vi "Bug2Test.vi"() -> ()   [LabVIEW 2013]
doc: "This example continually replans a path from Start to Goal while following the best known path, including through obstacles if necessary.\nThe Anytime D* search algorithm is useful when the world or the robot's understanding of the world is changing. Anytime D* maintains more information than the A* search algorithm so the robot can backtrack and find a new path more easily if it discovers the original path will not work."
panel:
  in  "Loop Time":u32=100
  out "Current Y":i32
  out "Current X":i32
  in  "y Goal":i32
  in  "x Goal":i32
  in  "Random Obstacles?":bool
  in  "% Random Obstacles":dbl=40.0 min=0.0 max=100.0 step=1.0 format="%#_3g"
  out "path on obstacles":dbl[][](graph)
  in  "y start":i32
  in  "x start":i32
  # "Configuration"
  # "X"
  # "Y"
  # "Start"
  # "X"
  # "Y"
  # "Goal"
  # "1) Choose the Start and Goal location and the % Random Obstacles.\n2) Run the VI.\n3) Adjust the controls in the Run-time Controls section to see the \n     effect each option has on path planning\n4) Change the Run Mode to Single Step to pause after each time\n the AD* VI runs"
  # "Robot"
  # "Obstacle"
  # "Unknown"
  # "Free"
  # "Path"
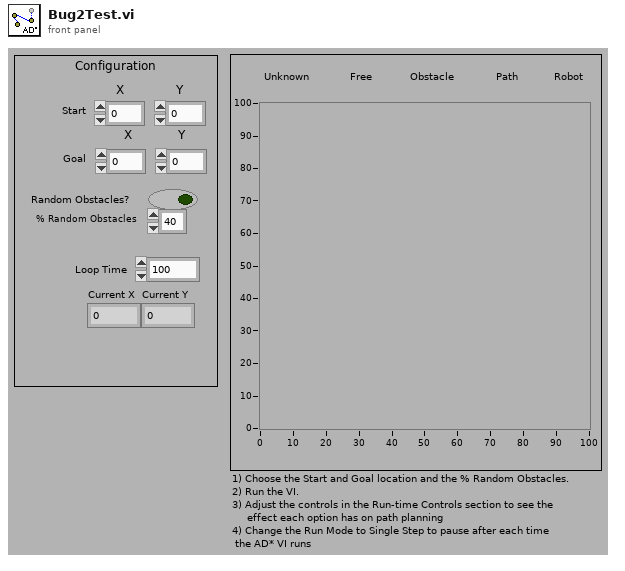
[diagram p1: front panel]
types:
  T1 = cluster{"x start":i32, "y start":i32, "x Goal":i32, "y Goal":i32}
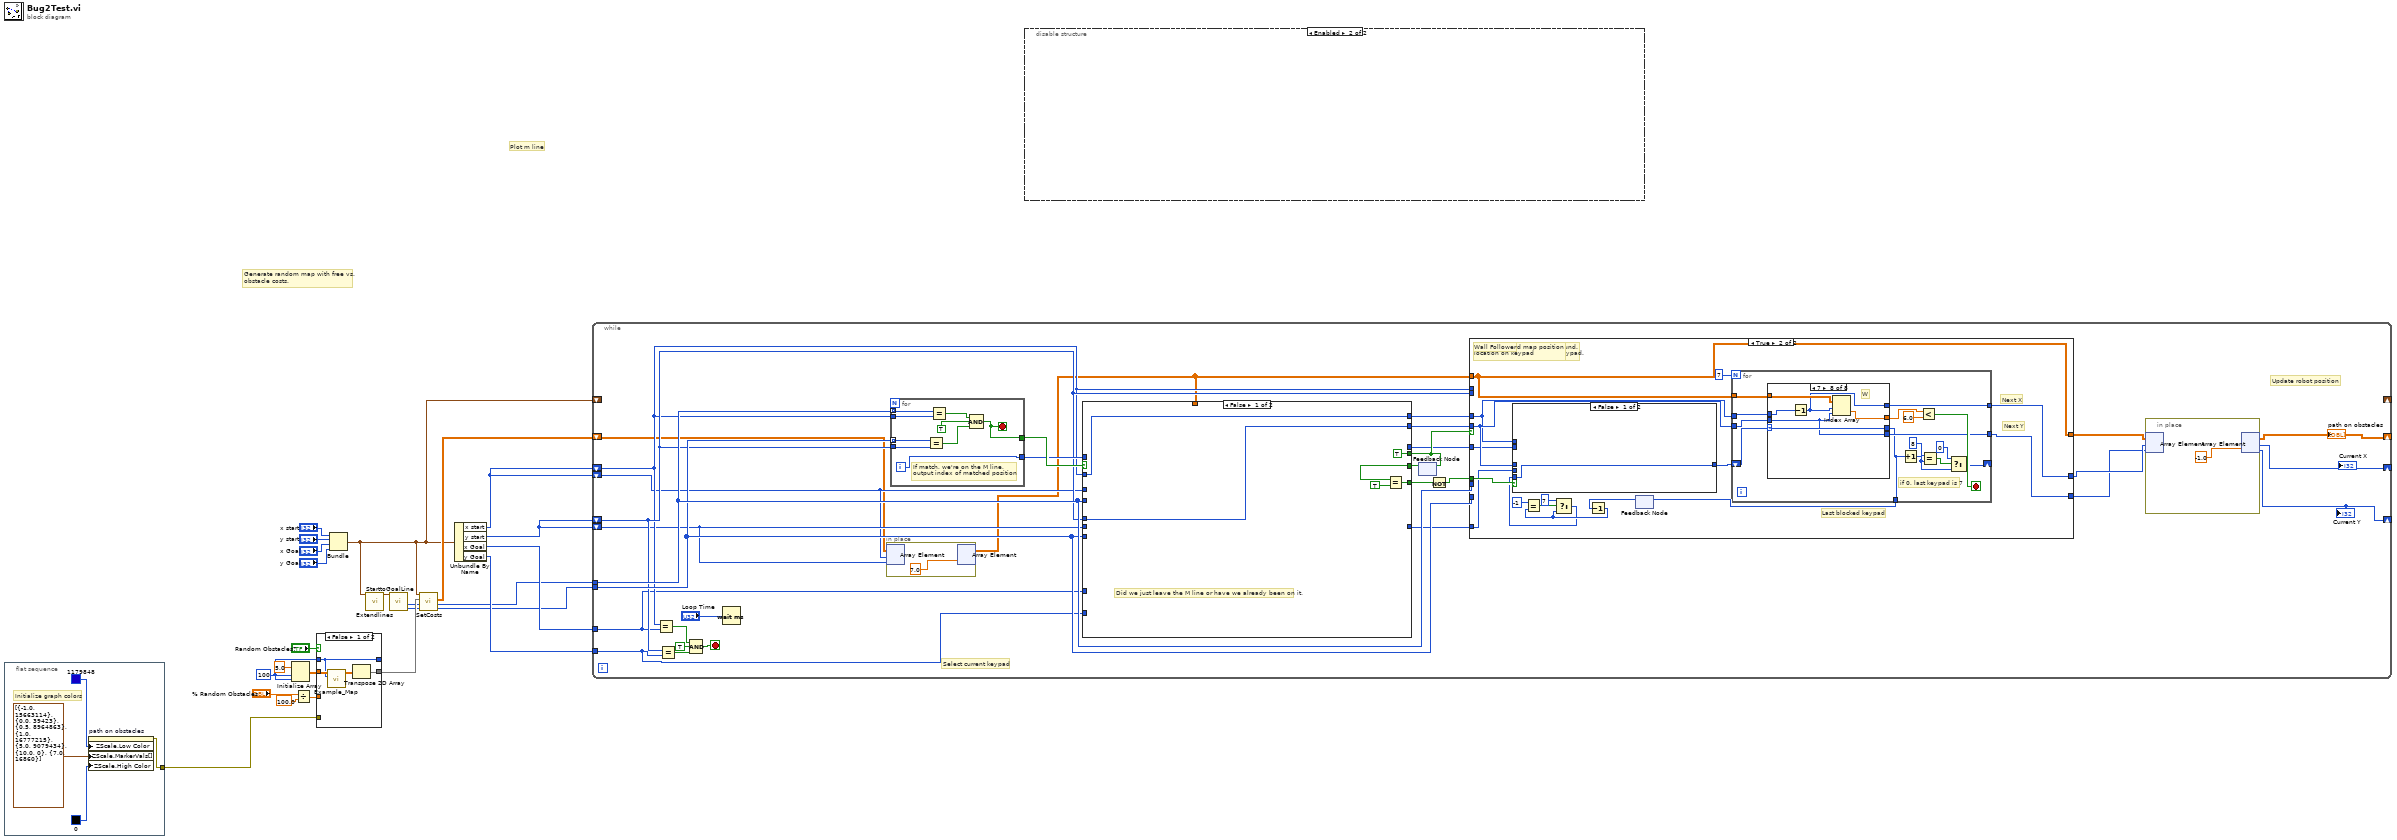
[diagram p0: block diagram]
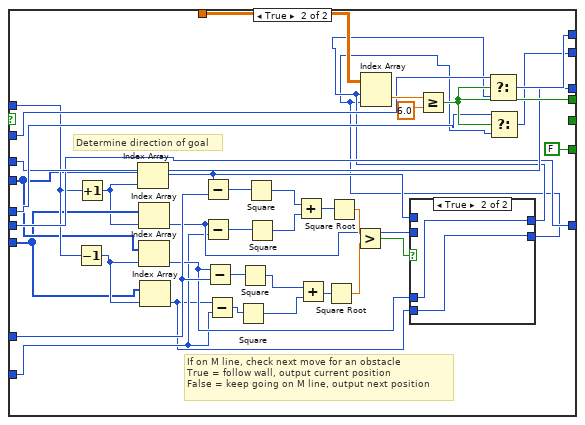
[diagram p2: hidden frame]
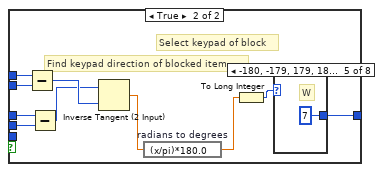
[diagram p5: hidden frame]
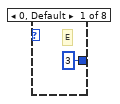
[diagram p6: hidden frame]
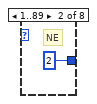
[diagram p7: hidden frame]
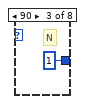
[diagram p8: hidden frame]
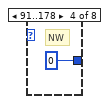
[diagram p9: hidden frame]
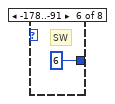
[diagram p10: hidden frame]
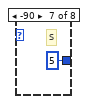
[diagram p11: hidden frame]
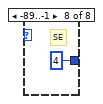
[diagram p12: hidden frame]
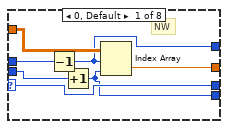
[diagram p13: hidden frame]
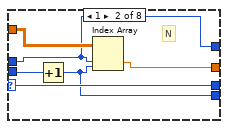
[diagram p14: hidden frame]
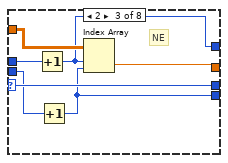
[diagram p15: hidden frame]
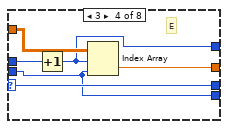
[diagram p16: hidden frame]
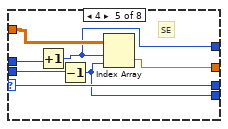
[diagram p17: hidden frame]
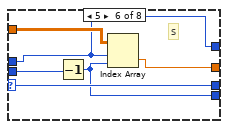
[diagram p18: hidden frame]
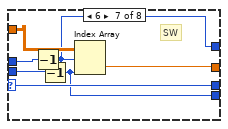
[diagram p19: hidden frame]
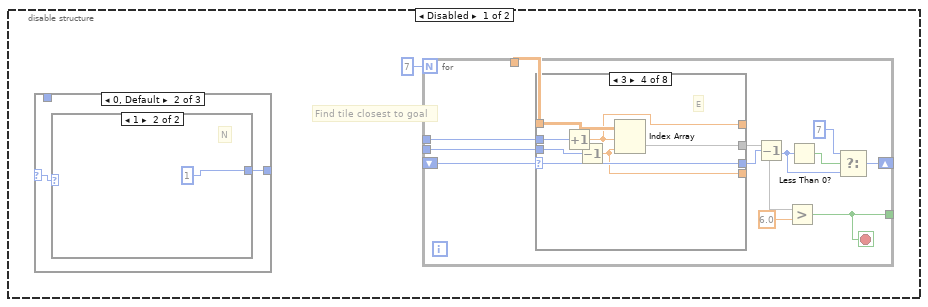
[diagram p20: hidden frame]
diagram:
  w21 = 100 ("dimension size")
  # "Plot m line"
  # "Generate random map with free vs.\nobstacle costs."
  n1 = flat-sequence {
    tunnel: [w25] -> w17
    frame #0 {
      # "Initialize graph colors"
      n2 = property on="path on obstacles" class="IntGraph (strict)"("ZScale.Low Color"=u32 1179848, "ZScale.MarkerVals[]"=cluster{dbl, u32}[] [{-1.0, 15663114}, {0.0, 39423}, {0.5, 8964863}, {1.0, 16777215}, {5.0, 9079434}, {10.0, 0}, {7.0, 16860}], "ZScale.High Color"=u32 0) -> (error out=w25:errorcluster)  [unwired: 2 in, 1 out]
    }
  }
  n3 = Initialize Array(5.0 ("\"unknown\" value for map"), w21, w21) -> (w18:dbl[][])
  n4 = Divide(x="% Random Obstacles", y=100.0) -> (x/y=w19:dbl)
  n5 = case shown="False" "Random Obstacles?" {
    tunnel: w19 -> [_ w36]
    tunnel: w18 -> [w32 w35]
    tunnel: [w29 w34] -> w14
    tunnel: w21 -> [w31 w33]
    tunnel: [w31 w33] -> _
    tunnel: w17 -> [_ _]
    frame False {
      n6 = call "Example_Map.vi"("dimension size"=w31, "Array in"=w32) -> ("Array out"=w30:dbl[][])  [unwired: 9 in]
      n7 = Transpose 2D Array(2D array=w30) -> (transposed array=w29:dbl[][])
    }
    frame True {
      n8 = call "Generate Random Obstacles.vi"("obstacle cost"=1000.0, "free cost"=2.0, "chance"=w36, "cost in"=w35) -> ("cost out"=w34:dbl[][])  [unwired: 7 in]
    }
  }
  n9 = Bundle("x start"="x start", "y start"="y start", "x Goal"="x Goal", "y Goal"="y Goal") -> (w1:T1)  [unwired: 1 in]
  n10 = call "Extendlines.vi"("StartGoalInfo"=w1) -> ("startgoal_calcout"=w16:cluster{"x0":i32, "x1":i32, "y1":i32, "y0":i32})  [unwired: 10 in]
  n11 = call "StarttoGoalLine.vi"("startgoal_calcout"=w16) -> ("y Line coords"=w3:i32[], "x Line coords"=w5:i32[])  [unwired: 9 in]
  n12 = call "SetCosts.vi"("y Line coords"=w3, "x Line coords"=w5, "cost in"=w14, "StartGoalInfo"=w1) -> ("y Line coords out"=w2:i32[], "x Line coords out"=w4:i32[], "cost out 2"=w13:dbl[][])  [unwired: 5 in]
  n13 = Unbundle By Name(w1) -> ("x start"=w12:i32, "y start"=w10:i32, "x Goal"=w7:i32, "y Goal"=w6:i32)
  n14 = while {
    shift-right: [w47] -> _
    shift-left: w12 -> [w52]
    shift-right: [w46] -> _
    shift-left: w10 -> [w53]
    tunnel: w4 -> [w68]
    tunnel: w2 -> [w63]
    shift-left: w12 -> [w42]
    shift-left: w10 -> [w43]
    tunnel: w7 -> [w45]
    tunnel: w6 -> [w44]
    shift-right: [w40] -> _
    shift-left: w13 -> [w39]
    shift-right: _ -> [_]
    shift-left: w1 -> [_]
    stop <- w51 stop-if-true
    # "Update robot position"
    # "Select current keypad"
    n15 = Equal?(x=w52, y=w45) -> (x = y?=w56:bool)
    n16 = Equal?(x=w53, y=w44) -> (x = y?=w55:bool)
    n17 = Compound Arithmetic op=AND(w56, TRUE ("value"), w55) -> (w51:bool)
    n18 = Wait (ms)(milliseconds to wait="Loop Time") -> ()  [unwired: 1 out]
    n19 = in-place {
      n20 = in-place-array #1(w39, w42, w43) -> ()  [unwired: 1 out]
      n21 = in-place-array #1(7.0) -> (w41:dbl[][])  [unwired: 2 out]
    }
    n22 = for {
      tunnel: w68 -> [w127] mode=indexing
      tunnel: w63 -> [w126] mode=indexing
      tunnel: w52 -> [w125]
      tunnel: w53 -> [w124]
      tunnel: [w120] -> w69
      tunnel: [w119] -> w65
      i -> [w119]
      stop <- w120 stop-if-true
      # "If match, we're on the M line,\noutput index of matched position"
      n23 = Equal?(x=w126, y=w124) -> (x = y?=w121:bool)
      n24 = Equal?(x=w127, y=w125) -> (x = y?=w123:bool)
      n25 = Compound Arithmetic op=AND(w123, TRUE ("y"), w121) -> (w120:bool)
    }
    n26 = feedback #2() -> (w61:bool)  [unwired: 1 in]
    n27 = case shown="False" w69 {
      tunnel: w63 -> [_ w100]
      tunnel: w68 -> [_ w102]
      tunnel: w41 -> [_ w114]
      tunnel: w52 -> [w73 w107]
      tunnel: w53 -> [w72 w106]
      tunnel: [TRUE w110] -> w62
      tunnel: [w73 w109] -> w67
      tunnel: [w72 w108] -> w66
      tunnel: w65 -> [_ w103]
      tunnel: w61 -> [w77 _]
      tunnel: [w75 FALSE] -> w60
      tunnel: w42 -> [_ w105]
      tunnel: w43 -> [_ w104]
      tunnel: [_ w105] -> w58
      tunnel: [_ w104] -> w57
      tunnel: w45 -> [_ w98]
      tunnel: w44 -> [_ w82]
      frame False {
        # "Did we just leave the M line or have we already been on it."
        n28 = Equal?(x=w77, y=TRUE) -> (x = y?=w75:bool)
      }
      frame True {
        # "Determine direction of goal"
        # "If on M line, check next move for an obstacle\nTrue = follow wall, output current position\nFalse = keep going on M line, output next position"
        n29 = Decrement(x=w103) -> (x-1=w101:i32)
        n30 = Increment(x=w103) -> (x+1=w99:i32)
        n31 = Index Array(array=w102, index=w99) -> (element=w85:i32)
        n32 = Index Array(array=w100, index=w99) -> (element=w84:i32)
        n33 = Index Array(array=w102, index=w101) -> (element=w83:i32)
        n34 = Index Array(array=w100, index=w101) -> (element=w80:i32)
        n35 = Subtract(x=w85, y=w98) -> (x-y=w97:i32)
        n36 = Subtract(x=w84, y=w82) -> (x-y=w96:i32)
        n37 = Subtract(x=w83, y=w98) -> (x-y=w95:i32)
        n38 = Subtract(x=w80, y=w82) -> (x-y=w94:i32)
        n39 = Square(x=w94) -> (x^2=w90:i32)
        n40 = Square(x=w95) -> (x^2=w91:i32)
        n41 = Square(x=w97) -> (x^2=w93:i32)
        n42 = Square(x=w96) -> (x^2=w92:i32)
        n43 = Add(x=w93, y=w92) -> (x+y=w89:i32)
        n44 = Add(x=w91, y=w90) -> (x+y=w88:i32)
        n45 = Square Root(x=w88) -> (sqrt(x)=w81:dbl)
        n46 = Square Root(x=w89) -> (sqrt(x)=w87:dbl)
        n47 = Greater?(x=w87, y=w81) -> (0:w86:bool)
        n48 = case shown="True" w86 {
          tunnel: w85 -> [w116 _]
          tunnel: w84 -> [w115 _]
          tunnel: w83 -> [_ w118]
          tunnel: w80 -> [_ w117]
          tunnel: [w116 w118] -> w79
          tunnel: [w115 w117] -> w78
          frame False {
          }
          frame True {
          }
        }
        n49 = Index Array(array=w114, index (row)=w79, index (col)=w78) -> (element=w113:dbl)
        n50 = Greater Or Equal?(x=w113, y=6.0) -> (x >= y?=w110:bool)
        n51 = Select(t=w107, s=w110, f=w79) -> (s? t:f=w109:i32)
        n52 = Select(t=w106, s=w110, f=w78) -> (s? t:f=w108:i32)
      }
    }
    n53 = feedback-in #2(w62) -> ()
    n54 = Not(x=w60) -> (.not. x?=w59:bool)
    n55 = case shown="True" w62 {
      tunnel: w41 -> [w128 w134]
      tunnel: w52 -> [_ _]
      tunnel: w53 -> [_ _]
      tunnel: w63 -> [_ _]
      tunnel: w68 -> [_ _]
      tunnel: [w128 w134] -> w50
      tunnel: w67 -> [w129 w133]
      tunnel: w66 -> [w130 w146]
      tunnel: [w129 w145] -> w49
      tunnel: [w130 w144] -> w48
      tunnel: w59 -> [_ w142]
      tunnel: w58 -> [_ w132]
      tunnel: w57 -> [_ w135]
      frame False {
        # "Next Position"
        # "update map with robot position"
        # "At this point, we're already on the M line, so we need \nto simply output the next M line point and iterate."
        # "M line follow"
      }
      frame True {
        # "Last blocked keypad"
        # "Next Y"
        # "Next X"
        # "Search until an opening is found.\nSave last value of blocked keypad."
        # "Output blocked map position\nlocation on keypad"
        # "Wall Follower"
        n56 = feedback #3() -> (w141:i32)  [unwired: 1 in]
        n57 = Decrement(x=w141) -> (x-1=w137:i32)
        n58 = Equal?(x=-1, y=w137) -> (x = y?=w139:bool)
        n59 = Select(t=7, s=w139, f=w137) -> (s? t:f=w136:i32)
        n60 = case shown="False" w142 {
          tunnel: w135 -> [_ w150]
          tunnel: w133 -> [_ w151]
          tunnel: [w148 w156] -> w143
          tunnel: w132 -> [_ w152]
          tunnel: w146 -> [_ w149]
          tunnel: w136 -> [w148 _]
          frame False {
          }
          frame True {
            # "Select keypad of block"
            # "Find keypad direction of blocked item"
            n61 = Subtract(x=w151, y=w152) -> (x-y=w158:i32)
            n62 = Subtract(x=w149, y=w150) -> (x-y=w157:i32)
            n63 = Inverse Tangent (2 Input)(1:w158, 2:w157) -> (0:w155:dbl)
            n64 = expression code="(x/pi)*180.0" "radians to degrees"(w155) -> (w154:dbl)
            n65 = To Long Integer(number=w154) -> (32bit integer=w153:i32)
            n66 = case shown="-180, -179, 179, 180" w153 {
              tunnel: [3 2 1 0 7 6 5 4] -> w156
              frame 0, Default {
                # "E"
              }
              frame 1..89 {
                # "NE"
              }
              frame 90 {
                # "N"
              }
              frame 91..178 {
                # "NW"
              }
              frame -180, -179, 179, 180 {
                # "W"
              }
              frame -178..-91 {
                # "SW"
              }
              frame -90 {
                # "S"
              }
              frame -89..-1 {
                # "SE"
              }
            }
          }
        }
        n67 = for {
          N: 7 -> [_]
          tunnel: w134 -> [w180]
          shift-right: [w172] -> _
          shift-left: w143 -> [w181]
          tunnel: w133 -> [w179]
          tunnel: w146 -> [w178]
          tunnel: [w174] -> w145
          tunnel: [w173] -> w144
          tunnel: [w167] -> w131
          stop <- w175 stop-if-true
          # "if 0, last keypad is 7"
          n68 = case shown="7" w181 {
            selector: w181 -> [w188 w194 w201 w207 w214 w220 w227 w233]
            tunnel: w180 -> [w187 w193 w200 w206 w213 w219 w226 w232]
            tunnel: [w188 w194 w201 w207 w214 w220 w227 w233] -> w167
            tunnel: w179 -> [w186 w190 w198 w204 w212 w216 w225 w231]
            tunnel: w178 -> [w185 w191 w196 w202 w211 w218 w224 w228]
            tunnel: [w184 w192 w199 w205 w210 w217 w223 w230] -> w177
            tunnel: [w183 w190 w197 w203 w209 w216 w222 w229] -> w174
            tunnel: [w182 w189 w195 w202 w208 w215 w221 w228] -> w173
            frame 0, Default {
              # "NW"
              n69 = Decrement(x=w186) -> (x-1=w183:i32)
              n70 = Increment(x=w185) -> (x+1=w182:i32)
              n71 = Index Array(array=w187, index (row)=w183, index (col)=w182) -> (element=w184:dbl)
            }
            frame 1 {
              # "N"
              n72 = Increment(x=w191) -> (x+1=w189:i32)
              n73 = Index Array(array=w193, index (row)=w190, index (col)=w189) -> (element=w192:dbl)
            }
            frame 2 {
              # "NE"
              n74 = Increment(x=w198) -> (x+1=w197:i32)
              n75 = Increment(x=w196) -> (x+1=w195:i32)
              n76 = Index Array(array=w200, index (row)=w197, index (col)=w195) -> (element=w199:dbl)
            }
            frame 3 {
              # "E"
              n77 = Increment(x=w204) -> (x+1=w203:i32)
              n78 = Index Array(array=w206, index (row)=w203, index (col)=w202) -> (element=w205:dbl)
            }
            frame 4 {
              # "SE"
              n79 = Increment(x=w212) -> (x+1=w209:i32)
              n80 = Decrement(x=w211) -> (x-1=w208:i32)
              n81 = Index Array(array=w213, index (row)=w209, index (col)=w208) -> (element=w210:dbl)
            }
            frame 5 {
              # "S"
              n82 = Decrement(x=w218) -> (x-1=w215:i32)
              n83 = Index Array(array=w219, index (row)=w216, index (col)=w215) -> (element=w217:dbl)
            }
            frame 6 {
              # "SW"
              n84 = Decrement(x=w225) -> (x-1=w222:i32)
              n85 = Decrement(x=w224) -> (x-1=w221:i32)
              n86 = Index Array(array=w226, index (row)=w222, index (col)=w221) -> (element=w223:dbl)
            }
            frame 7 {
              # "W"
              n87 = Decrement(x=w231) -> (x-1=w229:i32)
              n88 = Index Array(array=w232, index (row)=w229, index (col)=w228) -> (element=w230:dbl)
            }
          }
          n89 = Increment(x=w167) -> (x+1=w170:i32)
          n90 = Less?(x=w177, y=6.0) -> (x < y?=w175:bool)
          n91 = Equal?(x=8, y=w170) -> (x = y?=w171:bool)
          n92 = Select(t=0, s=w171, f=w170) -> (s? t:f=w172:i32)
        }
        n93 = feedback-in #3(w131) -> ()
      }
    }
    n94 = in-place {
      n95 = in-place-array #4(w50, w49, w48) -> ()  [unwired: 1 out]
      n96 = in-place-array #4(-1.0) -> (w40:dbl[][], w47:i32, w46:i32)
    }
    "path on obstacles" <- w40
    "Current X" <- w47
    "Current Y" <- w46
  }
  n97 = disable-structure shown="Enabled" {
    frame Disabled {
      # "Find tile closest to goal"
      n98 = case shown="0, Default" {
        selector: _ -> [w239 w244 _]
        tunnel: _ -> [_ _ w248]
        tunnel: [w238 w243 w247] -> _
        frame -1 {
          n99 = case shown="0, Default" w239 {
            tunnel: [u32 6 ("milliseconds to wait") u32 7 ("milliseconds to wait") u32 0 ("milliseconds to wait")] -> w238
            frame -1 {
              # "SE"
            }
            frame 0, Default {
              # "W"
            }
            frame 1 {
              # "NW"
            }
          }
        }
        frame 0, Default {
          n100 = case shown="1" w244 {
            tunnel: [u32 5 ("milliseconds to wait") u32 1 ("milliseconds to wait")] -> w243
            frame -1 {
              # "S"
            }
            frame 1 {
              # "N"
            }
          }
        }
        frame 1 {
          n101 = case shown="-1" w248 {
            tunnel: [u32 4 ("milliseconds to wait") u32 3 ("milliseconds to wait") u32 2 ("milliseconds to wait")] -> w247
            frame -1 {
              # "SE"
            }
            frame 0, Default {
              # "E"
            }
            frame 1 {
              # "NE"
            }
          }
        }
      }
      n102 = for {
        N: 7 -> [_]
        tunnel: _ -> [w263]
        tunnel: [w262] -> w234
        tunnel: [w261] -> w235
        shift-right: [w256] -> _
        shift-left: [w260] -> w236
        tunnel: [w252] -> _
        stop <- w252 stop-if-true
        n103 = case shown="3" w260 {
          selector: w260 -> [w270 w276 w282 w289 w296 w302 w309 w315]
          tunnel: w263 -> [w269 w275 w281 w288 w295 w301 w308 w314]
          tunnel: [w270 w276 w282 w289 w296 w302 w309 w315] -> w257
          tunnel: w262 -> [w268 w272 w279 w286 w294 w298 w307 w313]
          tunnel: w261 -> [w267 w273 w277 w285 w293 w300 w306 w310]
          tunnel: [w266 w274 w280 w287 w292 w299 w305 w312] -> w254
          tunnel: [w265 w272 w278 w284 w291 w298 w304 w311] -> _
          tunnel: [w264 w271 w277 w283 w290 w297 w303 w310] -> _
          frame 0, Default {
            # "NW"
            n104 = Decrement(x=w268) -> (x-1=w265:dbl)
            n105 = Increment(x=w267) -> (x+1=w264:dbl)
            n106 = Index Array(array=w269, index (row)=w265, index (col)=w264) -> (element=w266)
          }
          frame 1 {
            # "N"
            n107 = Increment(x=w273) -> (x+1=w271:dbl)
            n108 = Index Array(array=w275, index (row)=w272, index (col)=w271) -> (element=w274)
          }
          frame 2 {
            # "NE"
            n109 = Increment(x=w279) -> (x+1=w278:dbl)
            n110 = Index Array(array=w281, index (row)=w278, index (col)=w277) -> (element=w280)
          }
          frame 3 {
            # "E"
            n111 = Increment(x=w286) -> (x+1=w284:dbl)
            n112 = Decrement(x=w285) -> (x-1=w283:dbl)
            n113 = Index Array(array=w288, index (row)=w284, index (col)=w283) -> (element=w287)
          }
          frame 4 {
            # "SE"
            n114 = Increment(x=w294) -> (x+1=w291:dbl)
            n115 = Decrement(x=w293) -> (x-1=w290:dbl)
            n116 = Index Array(array=w295, index (row)=w291, index (col)=w290) -> (element=w292)
          }
          frame 5 {
            # "S"
            n117 = Decrement(x=w300) -> (x-1=w297:dbl)
            n118 = Index Array(array=w301, index (row)=w298, index (col)=w297) -> (element=w299)
          }
          frame 6 {
            # "SW"
            n119 = Decrement(x=w307) -> (x-1=w304:dbl)
            n120 = Decrement(x=w306) -> (x-1=w303:dbl)
            n121 = Index Array(array=w308, index (row)=w304, index (col)=w303) -> (element=w305)
          }
          frame 7 {
            # "W"
            n122 = Decrement(x=w313) -> (x-1=w311:dbl)
            n123 = Index Array(array=w314, index (row)=w311, index (col)=w310) -> (element=w312)
          }
        }
        n124 = Decrement(x=w257) -> (x-1=w259:u32)
        n125 = Greater?(x=w254, y=6.0) -> (0:w252:bool)
        n126 = Less Than 0?(x=w259) -> (x < 0?=w258:bool)
        n127 = Select(t=7, s=w258, f=w259) -> (s? t:f=w256:u32)
      }
    }
    frame Enabled {
    }
  }
